vi "Proces3_queue_datatype.vi"() -> (0 "output cluster":T1)   [LabVIEW 2019]
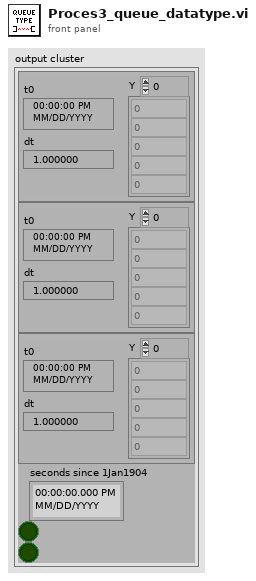
[diagram p1: front panel]
types:
  T1 = cluster{"Waveform":waveform(dbl), "Waveform":waveform(dbl), "Waveform":waveform(dbl), "seconds since 1Jan1904":timestamp, bool, bool}
  T2 = cluster{waveform(dbl), waveform(dbl), waveform(dbl), "seconds since 1Jan1904":timestamp, bool, bool}
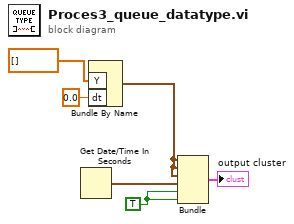
[diagram p0: block diagram]
diagram:
  w2 = TRUE
  n1 = Get Date/Time In Seconds() -> (seconds since 1Jan1904=w6:timestamp)
  n2 = Bundle By Name("Y"=dbl[] [], "dt"=0.0) -> (w3:waveform(dbl))  [unwired: 1 in]
  n3 = Bundle(w3, w3, w3, "seconds since 1Jan1904"=w6, w2, w2) -> (→"output cluster":T2)  [unwired: 1 in]
